vi "Straight Edge Detection1.vi"() -> ()   [LabVIEW 2014]
doc: "This example shows how to use Find Straight Edges in NI Vision. Find Straight Edges finds lines (or straight edges) within a search region. Find Straight Edges is a precursor function to many of the gauging and inspection tasks. For example, the location of the straight edges found within a region that encloses an object can interpreted as the boundaries of the object whose dimensions have to be measured for a gauging application or the presence of a crack in the surface of an object for an inspection application."
uses:
  <vilib>/vision/NI_Vision_Development_Module.lvlib
  <vilib>/vision/driver/NI_Vision_Acquisition_Software.lvlib
panel:
  in  "Camera Name":refnum<k21> caption="IMAQdx Session"
  out "Frame Rate":dbl(knob) scale=0.0..100.0
  out "采集视频":T1(plugin-control)
  out "Buffer Number":u32
  out "Numbers of lines(Red)":i32
  in  "Line Options":T2={"Number of Lines"=6, "Type"=4, "Minimum Score"=100.0, "Maximum Score"=1024.0, "Orientation"=0.0, "Angle Range"=10.0, "Angle Tolerance"=1.0, "Step Size"=3, "Min. SNR (db)"=0.0, "Min. Points (%)"=25.0, "Hough Iterations"=5} {"Min. Points (%)" min=0.0 max=100.0; "Min. SNR (db)" min=0.0; "Maximum Score" min=0.0 max=1024.0; "Minimum Score" min=1.0 max=1024.0 step=1.0; "Type" items=["First Edge Rake", "Best Edge Rake", "Hough Edge Rake", "First Edge Projection", "Best Edge Projection"]}
  in  "Edge Options":T3={"Edge Polarity"=0, "Kernel Size"=5, "Width"=3, "Minimum Edge Strength"=50.0, "Interpolation Type"=1, "Data Processing Method"=0} {"Data Processing Method" items=["Average", "Median"]; "Interpolation Type" items=["Zero Order"=0, "Bilinear"=1, "Bilinear Fixed"=4]; "Minimum Edge Strength" min=0.0 max=255.0 format="%.2g"; "Width" min=1 step=2; "Kernel Size" min=3 step=2; "Edge Polarity" items=["All Edges", "Rising Edges", "Falling Edges"]}
  in  "Search Direction":u32(ring) items=["Left to Right", "Right to Left", "Top to Bottom", "Bottom to Top"]
  out "边缘检测（右键单击图像Zoom to Fit还原图像）":T1(plugin-control)
  in  "Stop":bool
  # "使用说明\n1.点击CameraName选择摄像头；\n2.点击Search Direction选择需要检测的线型；\n3.点击检测工具条进行边缘检测。"
  # "功能介绍\n1.视频帧率设置Frame Rate；              4.线型参数设置Line Options；\n2.检测线型选择Search Direction；      5.检测工具条Test toolbar；\n3.边缘检测参数设置Edge Options；    6.检测结果数量显示Numbers of lines。"
  # "Test toolbar"
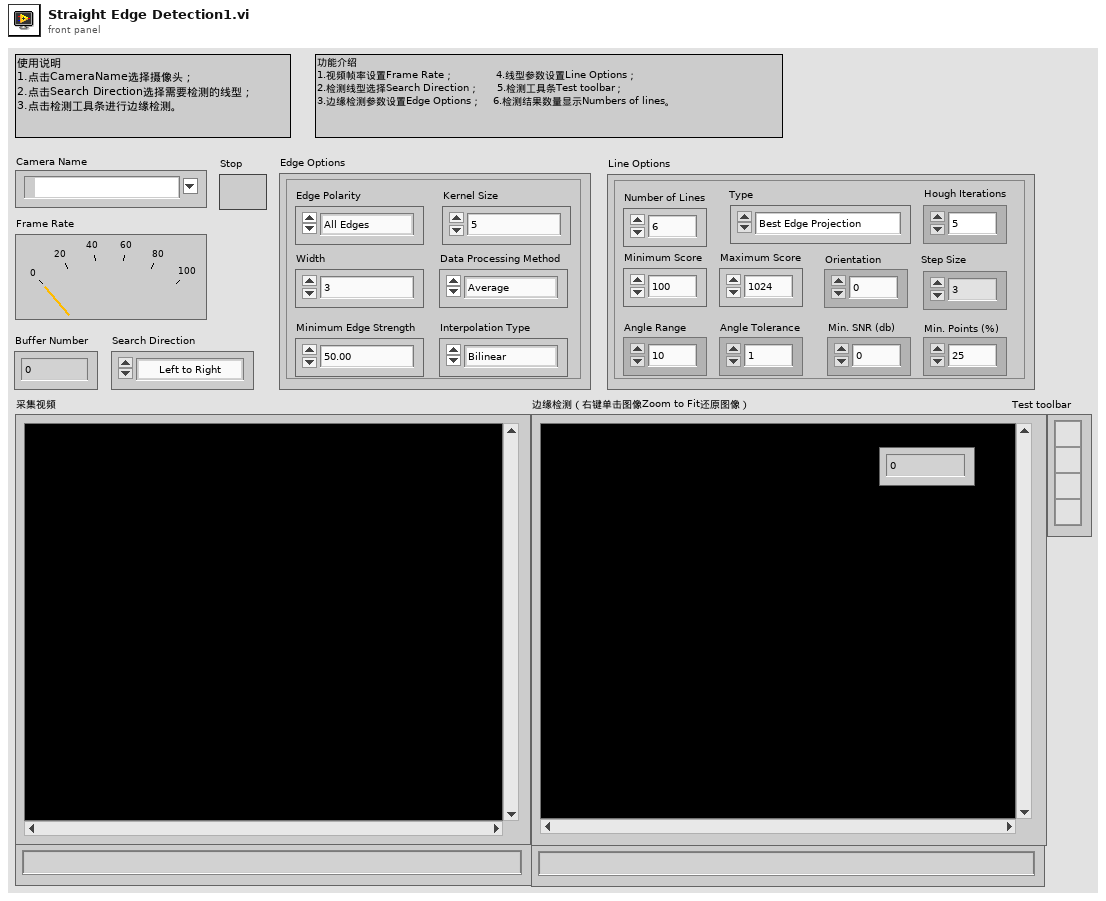
[diagram p1: front panel]
types:
  T1 = typedef "IMAQ Image.ctl" = refnum<image>
  T2 = cluster{"Number of Lines":i32, "Type":u16, "Minimum Score":dbl, "Maximum Score":dbl, "Orientation":dbl, "Angle Range":dbl, "Angle Tolerance":dbl, "Step Size":u32, "Min. SNR (db)":dbl, "Min. Points (%)":dbl, "Hough Iterations":i32}
  T3 = cluster{"Edge Polarity":u16, "Kernel Size":u32, "Width":u32, "Minimum Edge Strength":dbl, "Interpolation Type":u16, "Data Processing Method":u16}
  T4 = typedef "IMAQ Rectangle" = cluster{"Left":i32, "Top":i32, "Right":i32, "Bottom":i32, "Rotation":dbl}
  T5 = typedef "ROI Descriptor" = cluster{"Global Rectangle":i32[], "Contours":cluster{"ID":enum32{"External", "Internal"}, "Type":u32, "Coordinates":i32[]}[]}
  T6 = typedef "IMAQdx.ctl" = refnum<k21>
  T7 = cluster{"Global Rectangle":i32[], "Contours":cluster{"Contour Type":u32, "ROI Type":u32, "Points":i32[]}[]}
  T8 = cluster{"Point1 (Pixels)":cluster{"X":sgl, "Y":sgl}, "Point2 (Pixels)":cluster{"X":sgl, "Y":sgl}, "Point1 (Real-World)":cluster{"X":sgl, "Y":sgl}, "Point2 (Real-World)":cluster{"X":sgl, "Y":sgl}, "Angle (Pixel)":dbl, "Angle (Real-World)":dbl, "Score":dbl, "Straightness":dbl, "Average SNR (db)":dbl, "Calibration Valid":bool}[]
  T9 = typedef "Search Line.ctl" = cluster{"Start Point":cluster{"X":sgl, "Y":sgl}, "End Point":cluster{"X":sgl, "Y":sgl}, "Edge Info":T10[], "Edge Map":dbl[], "Calibration Valid":bool}
  T10 = typedef "Edge New.ctl" = cluster{"Location (Pixel)":cluster{"X":sgl, "Y":sgl}, "Location (Real-World)":cluster{"X":sgl, "Y":sgl}, "Distance (Pixel)":dbl, "Distance (Real-World)":dbl, "Strength":dbl, "Noise":dbl, "Rising?":bool}
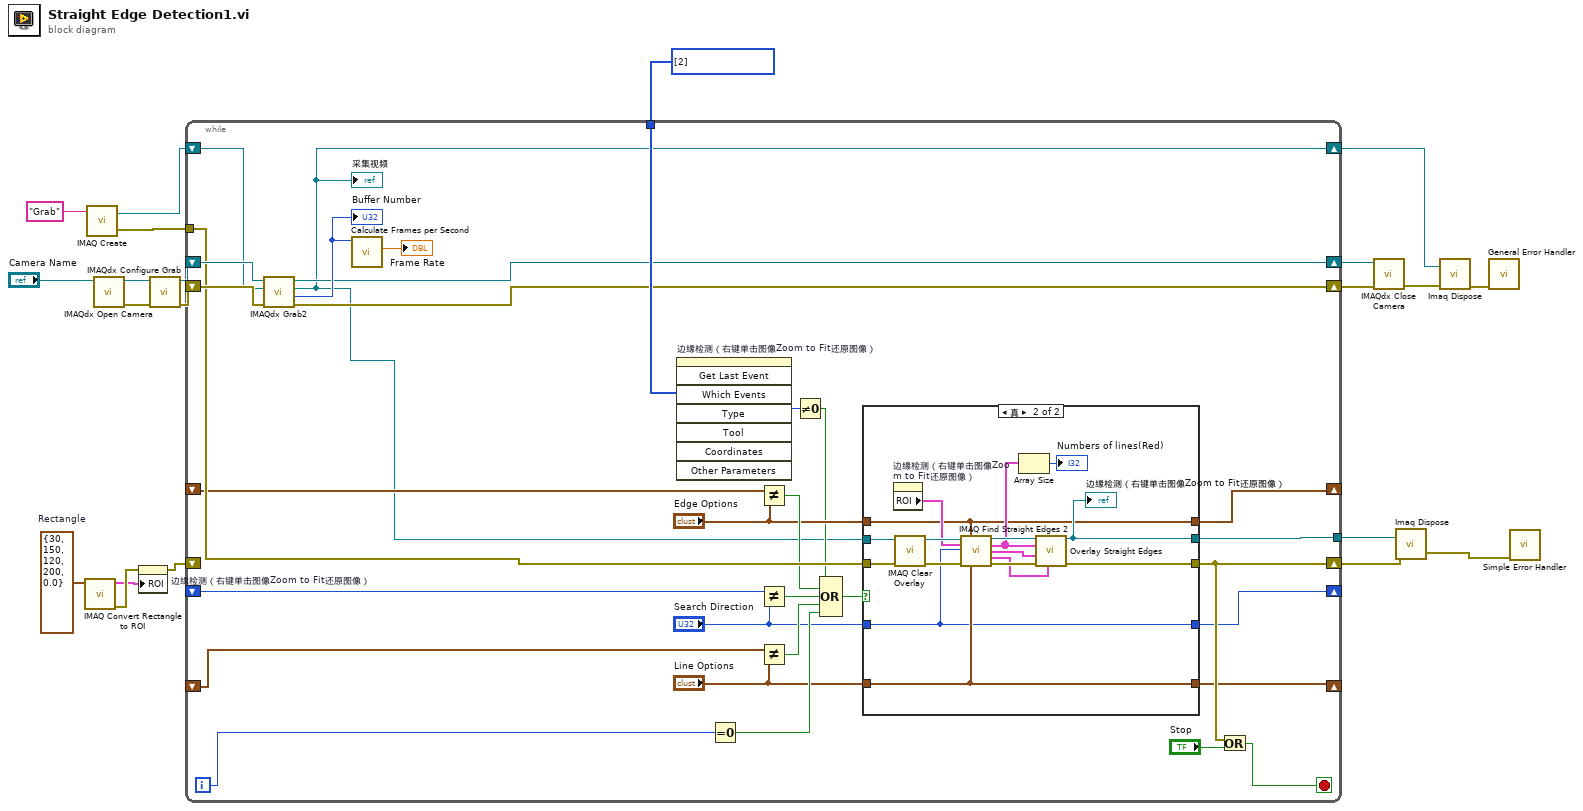
[diagram p0: block diagram]
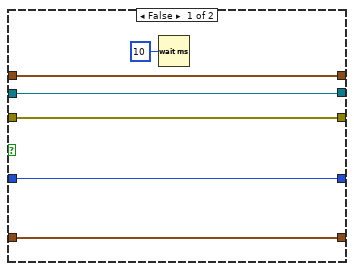
[diagram p2: hidden frame]
diagram:
  w19 = i32[] [2] items=["No Event"=0, "Click Event"=1, "Draw Event"=2, "Size Event"=4, "Scroll Event"=5, "Double Click Event"=8] ("Which Events")
  w20 = T4 {"Left"=30, "Top"=150, "Right"=120, "Bottom"=200, "Rotation"=0.0}  # Rectangle
  n1 = call "IMAQ Convert Rectangle to ROI"("Rectangle"=w20) -> ("error out"=w18:errorcluster, "ROI Descriptor"=w17:T5)  [unwired: 8 in]
  n2 = call "IMAQ Create"("Image Name"="Grab") -> ("New Image"=w1:T1, "error out"=w4:errorcluster)  [unwired: 3 in, 1 out]
  n3 = call <vilib>:"IMAQdx Open Camera.vi"("Session In"="Camera Name") -> ("error out"=w11:errorcluster, "Session Out"=w10:T6)  [unwired: 2 in, 7 out]
  n4 = property on="边缘检测（右键单击图像Zoom to Fit还原图像）" class="ImageControl"(error in=w18, "ROI"=w17) -> (error out=w16:errorcluster)  [unwired: 1 in, 1 out]
  n5 = call <vilib>:"IMAQdx Configure Grab.vi"("error in"=w11, "Session In"=w10) -> ("error out"=w14:errorcluster, "Session Out"=w15:T6)  [unwired: 8 out]
  n6 = while {
    tunnel: w19 -> [w52]
    tunnel: w4 -> [w48]
    tunnel: [w46] -> w2
    shift-right: [w47] -> w3
    shift-left: w16 -> [_]
    shift-right: [w24] -> w13
    shift-left: w15 -> [w51]
    shift-right: [w23] -> w12
    shift-left: w14 -> [w50]
    shift-right: [w22] -> w8
    shift-left: w1 -> [w49]
    shift-right: [w32] -> _
    shift-left: _ -> [w31]
    shift-right: [w30] -> _
    shift-left: _ -> [w29]
    shift-right: [w28] -> _
    shift-left: _ -> [w27]
    i -> [w26]
    stop <- w25 stop-if-true
    n7 = call <vilib>:"IMAQdx Grab2.vi"("error in"=w50, "Image In"=w49, "Session In"=w51) -> ("error out"=w23:errorcluster, "Buffer Number Out"=w44:u32, "Image Out"=w22:T1, "Session Out"=w24:T6)  [unwired: 5 in]
    "采集视频" <- w22
    "Buffer Number" <- w44
    n8 = call <vilib>:"Calculate Frames per Second.vi"("Buffer Number"=w44) -> ("Processed Frames/s"=→"Frame Rate":dbl)  [unwired: 8 in, 2 out]
    n9 = invoke on="边缘检测（右键单击图像Zoom to Fit还原图像）" class="ImageControl" method="Get Last Event"("Which Events"=w52) -> ("Type"=w34:i32)  [unwired: 7 in, 7 out]
    n10 = Equal To 0?(x=w26) -> (x = 0?=w40:bool)
    n11 = Not Equal?(x=w27, y="Edge Options") -> (x != y?=w39:bool)
    n12 = Not Equal?(x=w29, y="Search Direction") -> (x != y?=w43:bool)
    n13 = Not Equal?(x=w31, y="Line Options") -> (x != y?=w41:bool)
    n14 = Not Equal To 0?(x=w34) -> (x != 0?=w33:bool)
    n15 = Compound Arithmetic op=OR(w33, w39, w43, w41, w40) -> (w42:bool)
    n16 = case shown="真" w42 {
      tunnel: w22 -> [w58 w74]
      tunnel: [w58 w73] -> w46
      tunnel: w48 -> [w57 w72]
      tunnel: [w57 w71] -> w47
      tunnel: "Edge Options" -> [w53 w59]
      tunnel: "Search Direction" -> [w55 w60]
      tunnel: "Line Options" -> [w56 w61]
      tunnel: [w56 w61] -> w32
      tunnel: [w55 w60] -> w30
      tunnel: [w53 w59] -> w28
      frame False {
        n17 = Wait (ms)(milliseconds to wait=u32 10) -> ()  [unwired: 1 out]
      }
      frame True {
        n18 = property on="边缘检测（右键单击图像Zoom to Fit还原图像）" class="ImageControl"() -> ("ROI"=w68:T7)  [unwired: 2 in, 2 out]
        n19 = call "IMAQ Clear Overlay"("error in (no error)"=w72, "Image"=w74) -> ("error out"=w70:errorcluster, "Image Out"=w69:T1)  [unwired: 8 in]
        n20 = call "IMAQ Find Straight Edges 2"("Image"=w69, "Edge Options"=w59, "ROI Descriptor"=w68, "Search Direction"=w60, "error in (no error)"=w70, "Line Options"=w61) -> ("Image (duplicate)"=w67:T1, "Straight Edges"=w63:T8, "Search Lines Information"=w66:T9[], "Used Edges"=w64:cluster{"Edge Information":T10[]}[], "error out"=w65:errorcluster)  [unwired: 5 in]
        n21 = Array Size(array=w63) -> (size(s)=→"Numbers of lines(Red)":i32)
        n22 = call "Overlay Straight Edges.vi"("All Edges (Pixel)"=w64, "error in"=w65, "Search Lines Information"=w66, "Straight Edges"=w63, "Image In"=w67) -> ("error out"=w71:errorcluster, "Image Out"=w73:T1)  [unwired: 5 in]
        "边缘检测（右键单击图像Zoom to Fit还原图像）" <- w73
      }
    }
    n23 = Or(x=w47, y="Stop") -> (x .or. y?=w25:bool)
  }
  n24 = call <vilib>:"IMAQdx Close Camera.vi"("error in"=w12, "Session In"=w13) -> ("error out"=w7:errorcluster)  [unwired: 9 out]
  n25 = call "Imaq Dispose"("Image"=w2, "error in (no error)"=w3) -> ("error out"=w21:errorcluster)  [unwired: 4 in]
  n26 = call "Imaq Dispose"("Image"=w8, "error in (no error)"=w7) -> ("error out"=w6:errorcluster)  [unwired: 4 in]
  n27 = call <vilib>:"General Error Handler.vi"("error in (no error)"=w6) -> ()  [unwired: 2 in, 13 out]
  n28 = call <vilib>:"Simple Error Handler.vi"("error in (no error)"=w21) -> ()  [unwired: 4 in, 5 out]
